vi "Feeder Control.vi"(4 "Collect from Feeder?":bool) -> ()   [LabVIEW 2012]
uses:
  BotStatus.vi
  Motors Values.vi
panel:
  out "Feeder Mode Enabled in Stack":bool
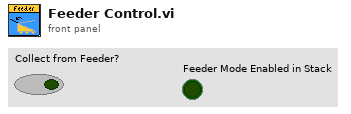
[diagram p1: front panel]
types:
  T1 = typedef "WPI_DigitalInputDevRef.ctl" = cluster{"DevStatus":errorcluster, "DIO Channel":T2, "Digital Module":T3}
  T2 = typedef "FPGA_DIOChannel.ctl" = enum8{"DIO 1", "DIO 2", "DIO 3", "DIO 4", "DIO 5", "DIO 6", "DIO 7", "DIO 8", "DIO 9", "DIO 10", "DIO 11", "DIO 12", "DIO 13", "DIO 14", "Invalid"}
  T3 = typedef "FPGA_TypedefDigitalModule.ctl" = enum16{"Digital Module 1", "Digital Module 2"}
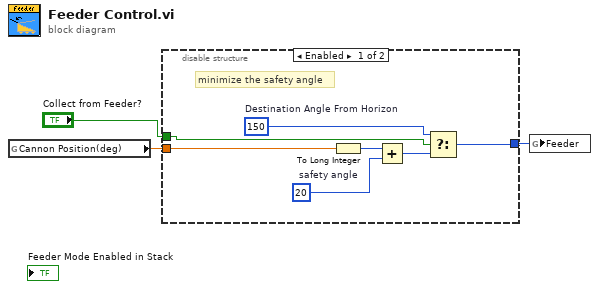
[diagram p0: block diagram]
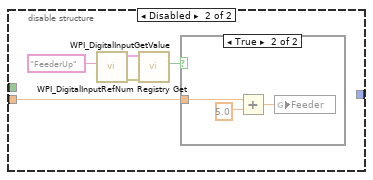
[diagram p2: hidden frame]
diagram:
  n1 = global read "BotStatus.vi" "Cannon Position(deg)"() -> (w3:dbl)
  n2 = disable-structure shown="Enabled" {
    disable-tunnel: w3 -> [w9 w11]
    disable-tunnel: "Collect from Feeder?" -> [w7 _]
    disable-tunnel: [w5 _] -> w1
    frame Enabled {
      w6 = 150  # Destination Angle From Horizon
      w10 = 20  # safety angle
      # "minimize the safety angle"
      n3 = To Long Integer(number=w9) -> (32bit integer=w4:i32)
      n4 = Add(x=w4, y=w10) -> (x+y=w8:i32)
      n5 = Select(t=w6, s=w7, f=w8) -> (s? t:f=w5:i32)
    }
    frame Disabled {
      n6 = call <vilib>:"WPI_DigitalInputRefNum Registry Get.vi"("refnum name"="FeederUp") -> ("error out"=w13:errorcluster, "DigitalInputDevRef"=w12:T1)  [unwired: 9 in]
      n7 = call <vilib>:"WPI_DigitalInputGetValue.vi"("error in (no error)"=w13, "DigitalInputDevRef"=w12) -> ("Value"=w15:bool)  [unwired: 7 in, 2 out]
      n8 = case shown="True" w15 {
        tunnel: w11 -> [_ w18]
        frame False {
        }
        frame True {
          n9 = Add(x=w18, y=5.0) -> (x+y=w16:dbl)
          n10 = global write "Motors Values.vi" "Feeder"(w16) -> ()
        }
      }
    }
  }
  n11 = global write "Motors Values.vi" "Feeder"(w1) -> ()
